vi "Dashboard custom_bartender.vi"() -> ()   [LabVIEW 2017]
uses:
  C:/Users/IMR Lab/Documents/LabVIEW Data/UniversalRobotsSDK_LABView/LabVIEW/Examples/LabVIEW10/UnderAutomation.UniversalRobots.dll
  UnderAutomation.UniversalRobots.dll
panel:
  out "\"3\"":bool
  out "\"2\"":bool
  out "\"1\"":bool
  out "UDP Loop Counter":i32
  out "UDP dataout":string
  in  "UDP":bool
  in  "stop":bool
  in  "TCP switch (server)":bool
  out "Rx":dbl
  out "Rz":dbl
  out "Ry":dbl
  out "Enabled":bool
  out "Port":i32
  in  "Move to particular posture":bool
  in  "Move to Zero position":bool
  out "Connected":bool
  in  "Robot IP(192.168.112.182)":string
  out "Connect error":errorcluster
  in  "Power on\nRelease brake":bool
  in  "Power off":bool
  in  "Connect":bool
  in  "Send script":bool
  in  "Script to execute":string
  out "Powered on":bool
  out "X":dbl
  out "Y":dbl
  out "Z":dbl
  out "License state":string
  # "movel(p[-0.0753945, -0.304532, 0.314608, -0.194623, 2.71667, -1.00228], a= 0.5, v=0.25)"
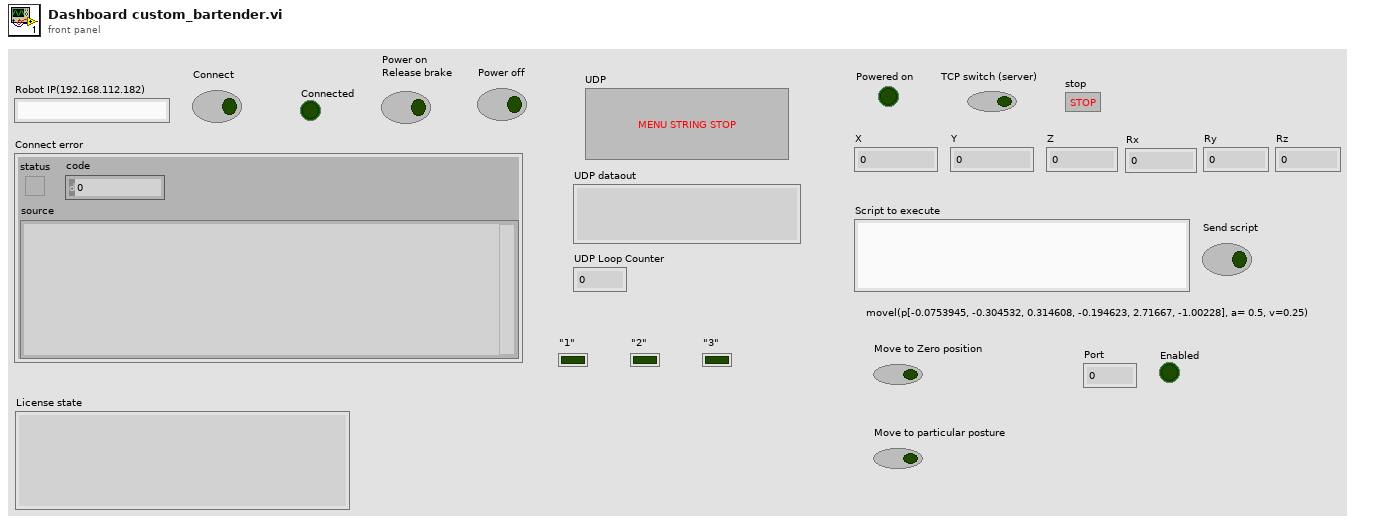
[diagram p1: front panel]
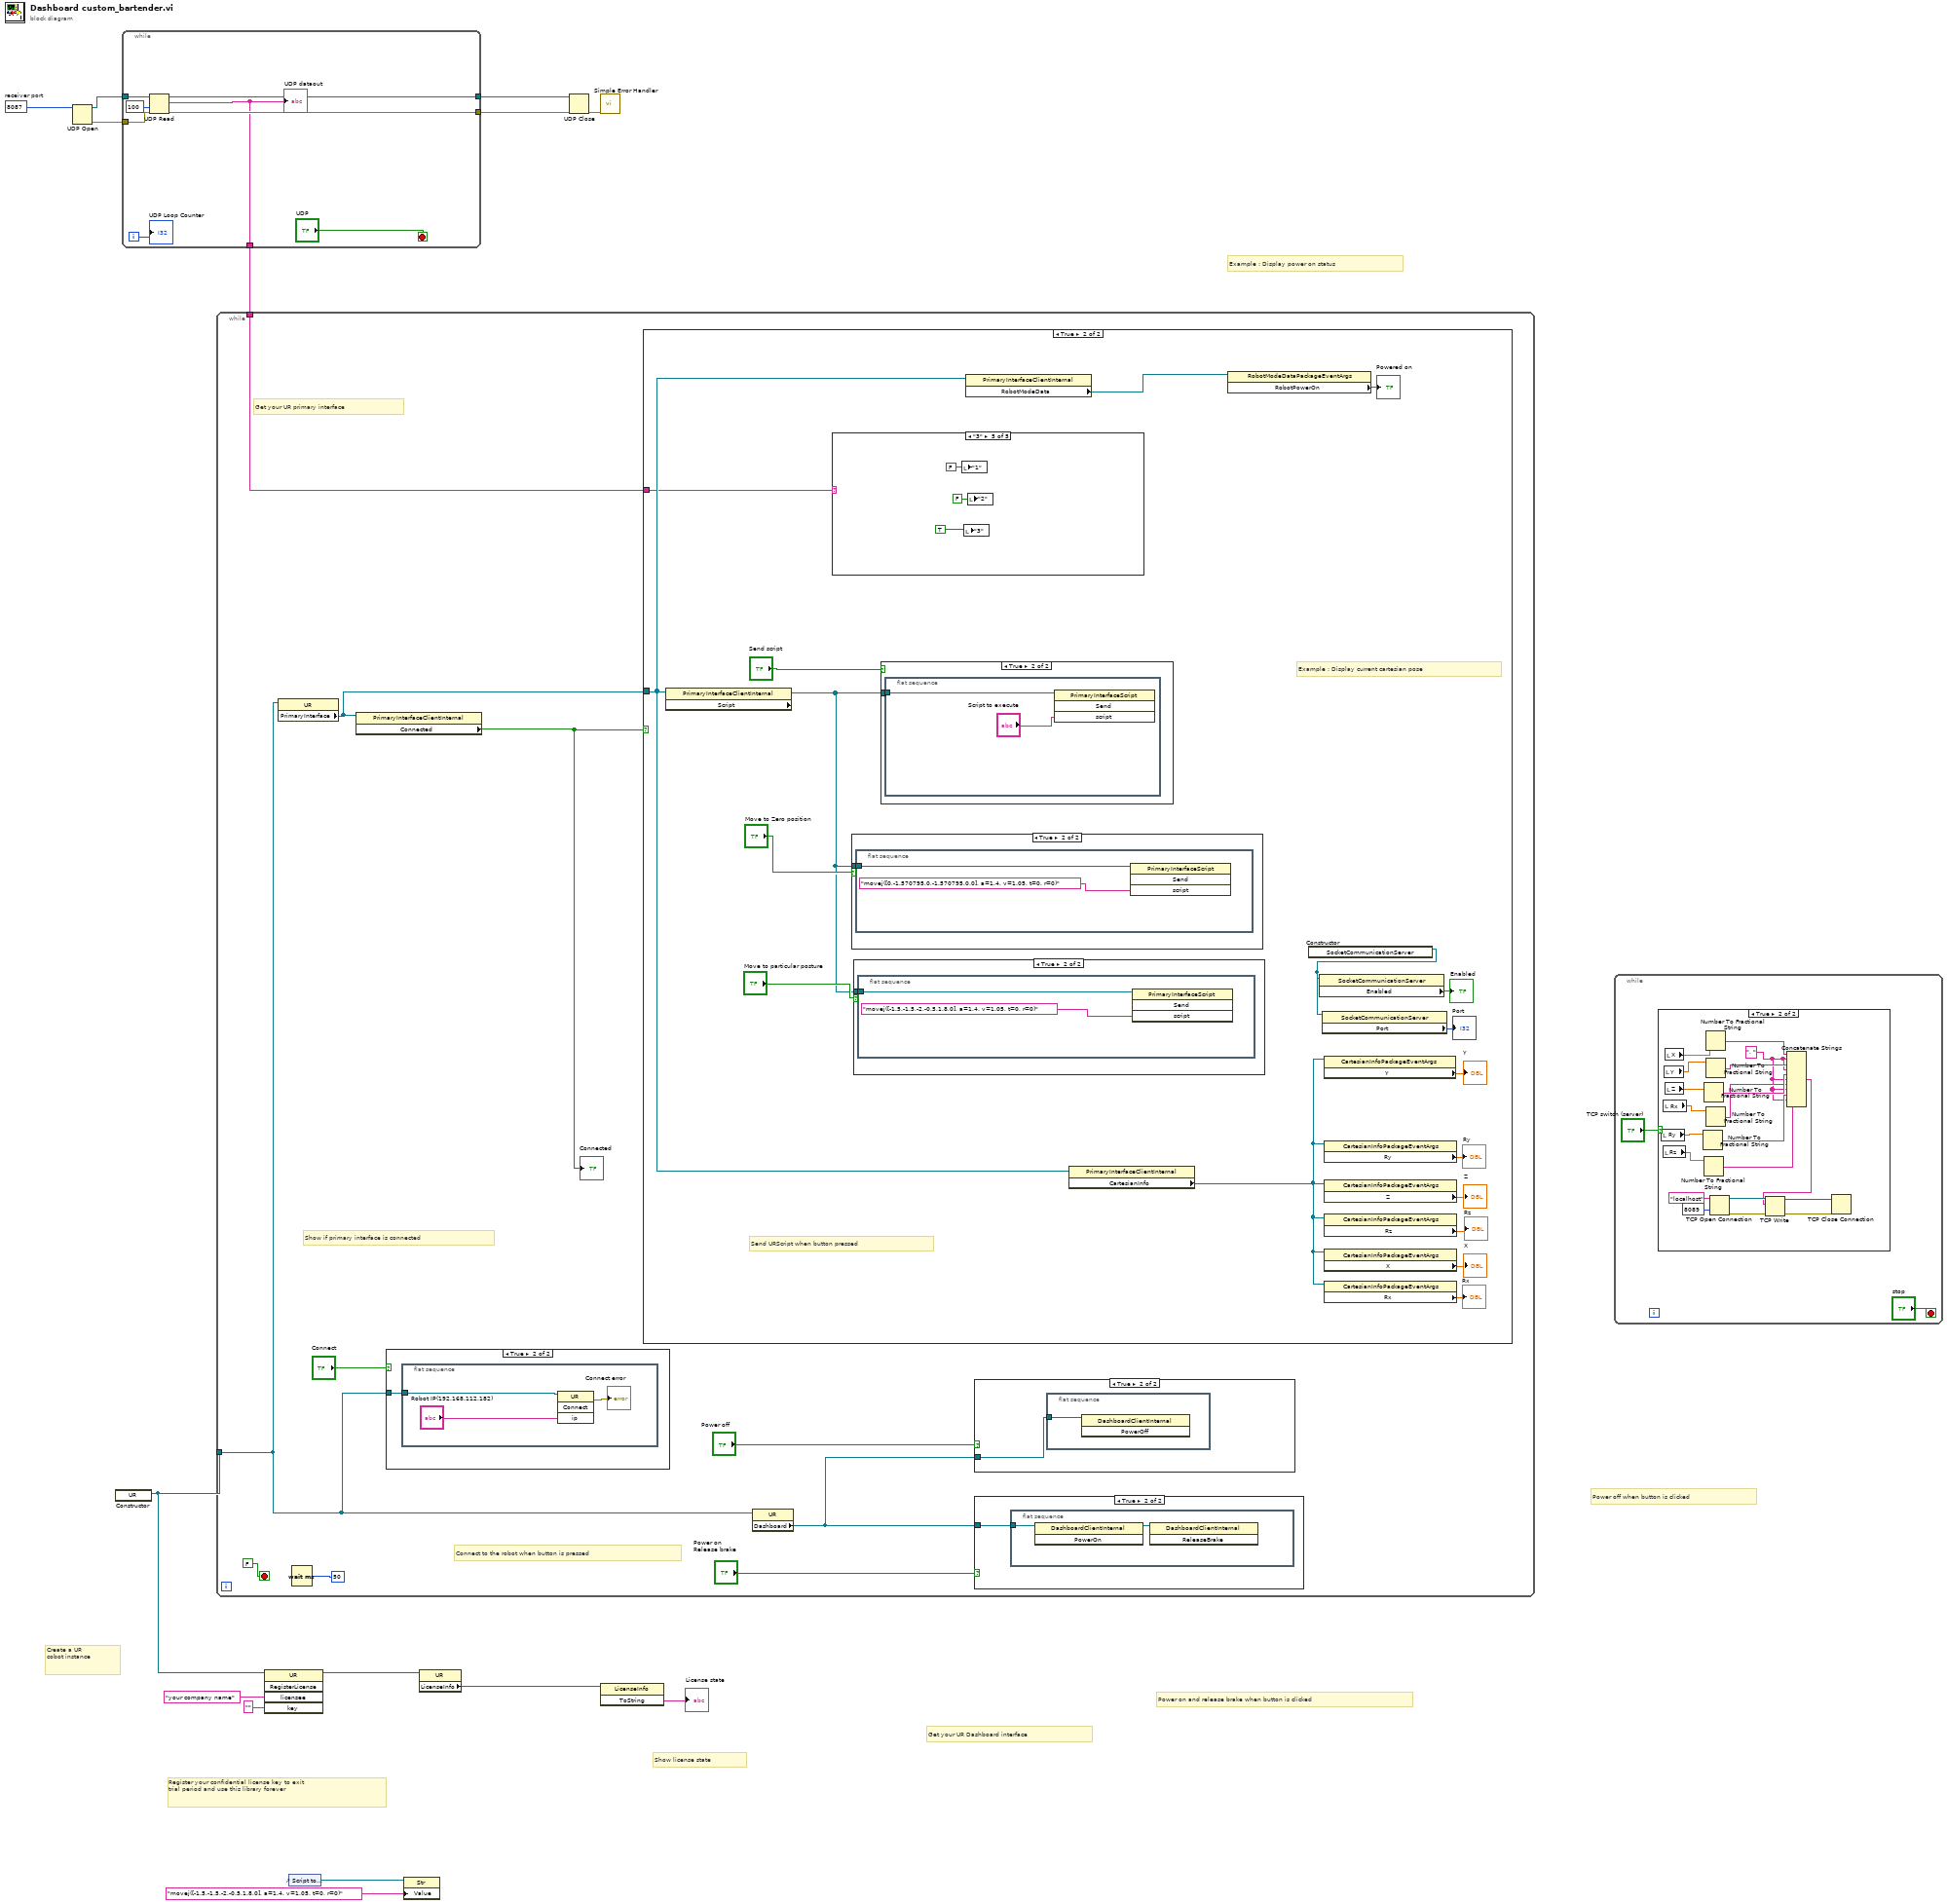
[diagram p0: block diagram]
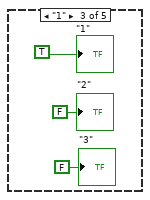
[diagram p6: hidden frame]
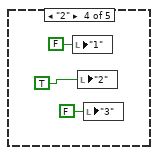
[diagram p7: hidden frame]
diagram:
  w7 = u16 8087  # receiver port
  # "Example : Display power on status"
  # "Create a UR\ncobot instance"
  # "Show license state"
  # "Register your confidential license key to exit\ntrial period and use this library forever"
  # "Power off when button is clicked"
  # "Power on and release brake when button is clicked"
  # "Get your UR Dashboard interface"
  n1 = UDP Open(11:w7) -> (port=w3:refnum<k16>, 0:w2:errorcluster)  [unwired: 4 in, 1 out]
  n2 = constructor class="UR"() -> (reference out=w10:refnum<k24>)  [unwired: 3 in, 2 out]
  n3 = while {
    tunnel: [w22] -> w5
    tunnel: [w21] -> w4
    tunnel: w3 -> [w20]
    tunnel: w2 -> [w19]
    tunnel: [w16] -> w1
    i -> [w18]
    stop <- "UDP" stop-if-true
    n4 = UDP Read(connection ID=w20, timeout ms (25000)=100, 8:w19) -> (data out=w16:string, error out=w21:errorcluster, 3:w22:refnum<k16>)  [unwired: 3 out]
    "UDP dataout" <- w16
    "UDP Loop Counter" <- w18
  }
  n5 = while {
    tunnel: w10 -> [w25]
    tunnel: w1 -> [w24]
    stop <- FALSE stop-if-true
    # "Connect to the robot when button is pressed"
    # "Show if primary interface is connected"
    # "Get your UR primary interface"
    n6 = property class="UR"(reference=w25) -> ("PrimaryInterface"=w28:refnum<k24>)  [unwired: 1 in, 2 out]
    n7 = Wait (ms)(milliseconds to wait=u32 50) -> ()  [unwired: 1 out]
    n8 = property class="PrimaryInterfaceClientInternal"(reference=w28) -> ("Connected"=w27:bool)  [unwired: 1 in, 2 out]
    "Connected" <- w27
    n9 = case shown="True" "Connect" {
      tunnel: w25 -> [_ w75]
      frame False {
      }
      frame True {
        n10 = flat-sequence {
          tunnel: w75 -> [w77]
          frame #0 {
            n11 = invoke class="UR" method="Connect"(reference=w77, "ip"="Robot IP(192.168.112.182)") -> (error out=→"Connect error":errorcluster)  [unwired: 2 in, 3 out]
          }
        }
      }
    }
    n12 = case shown="True" w27 {
      tunnel: w28 -> [_ w45]
      tunnel: w24 -> [_ w34]
      frame False {
      }
      frame True {
        # "Send URScript when button pressed"
        # "Example : Display current cartesian pose"
        n13 = property class="PrimaryInterfaceClientInternal"(reference=w45) -> ("Script"=w42:refnum<k24>)  [unwired: 1 in, 2 out]
        n14 = case shown="\"3\"" w34 {
          frame "False", Default {
          }
          frame "True" {
          }
          frame "1" {
            "\"1\"" <- TRUE
            "\"2\"" <- FALSE ("\"2\"")
            "\"3\"" <- FALSE ("\"3\"")
          }
          frame "2" {
            n15 = local write "\"1\""(FALSE ("\"1\"")) -> ()
            n16 = local write "\"2\""(TRUE) -> ()
            n17 = local write "\"3\""(FALSE ("\"3\"")) -> ()
          }
          frame "3" {
            n18 = local write "\"1\""(FALSE ("\"1\"")) -> ()
            n19 = local write "\"3\""(TRUE) -> ()
            n20 = local write "\"2\""(FALSE ("\"2\"")) -> ()
          }
        }
        n21 = case shown="True" "Move to Zero position" {
          tunnel: w42 -> [_ w64]
          frame False {
          }
          frame True {
            n22 = flat-sequence {
              tunnel: w64 -> [w66]
              frame #0 {
                n23 = invoke class="PrimaryInterfaceScript" method="Send"(reference=w66, "script"="movej([0,-1.570795,0,-1.570795,0,0], a=1.4, v=1.05, t=0, r=0)") -> ()  [unwired: 2 in, 4 out]
              }
            }
          }
        }
        n24 = case shown="True" "Move to particular posture" {
          tunnel: w42 -> [_ w61]
          frame False {
          }
          frame True {
            n25 = flat-sequence {
              tunnel: w61 -> [w63]
              frame #0 {
                n26 = invoke class="PrimaryInterfaceScript" method="Send"(reference=w63, "script"="movej([-1.5,-1.5,-2,-0.5,1.8,0], a=1.4, v=1.05, t=0, r=0)") -> ()  [unwired: 2 in, 4 out]
              }
            }
          }
        }
        n27 = case shown="True" "Send script" {
          tunnel: w42 -> [_ w67]
          frame False {
          }
          frame True {
            n28 = flat-sequence {
              tunnel: w67 -> [w69]
              frame #0 {
                n29 = invoke class="PrimaryInterfaceScript" method="Send"(reference=w69, "script"="Script to execute") -> ()  [unwired: 2 in, 4 out]
              }
            }
          }
        }
        n30 = property class="PrimaryInterfaceClientInternal"(reference=w45) -> ("RobotModeData"=w50:refnum<k24>)  [unwired: 1 in, 2 out]
        n31 = property class="PrimaryInterfaceClientInternal"(reference=w45) -> ("CartesianInfo"=w36:refnum<k24>)  [unwired: 1 in, 2 out]
        n32 = property class="RobotModeDataPackageEventArgs"(reference=w50) -> ("RobotPowerOn"=→"Powered on":bool)  [unwired: 1 in, 2 out]
        n33 = constructor class="SocketCommunicationServer"() -> (reference out=w41:refnum<k24>)  [unwired: 3 in, 2 out]
        n34 = property class="SocketCommunicationServer"(reference=w41) -> ("Enabled"=→"Enabled":bool)  [unwired: 1 in, 2 out]
        n35 = property class="SocketCommunicationServer"(reference=w41) -> ("Port"=→"Port":i32)  [unwired: 1 in, 2 out]
        n36 = property class="CartesianInfoPackageEventArgs"(reference=w36) -> ("Y"=→"Y":dbl)  [unwired: 1 in, 2 out]
        n37 = property class="CartesianInfoPackageEventArgs"(reference=w36) -> ("Ry"=→"Ry":dbl)  [unwired: 1 in, 2 out]
        n38 = property class="CartesianInfoPackageEventArgs"(reference=w36) -> ("Z"=→"Z":dbl)  [unwired: 1 in, 2 out]
        n39 = property class="CartesianInfoPackageEventArgs"(reference=w36) -> ("Rz"=→"Rz":dbl)  [unwired: 1 in, 2 out]
        n40 = property class="CartesianInfoPackageEventArgs"(reference=w36) -> ("X"=→"X":dbl)  [unwired: 1 in, 2 out]
        n41 = property class="CartesianInfoPackageEventArgs"(reference=w36) -> ("Rx"=→"Rx":dbl)  [unwired: 1 in, 2 out]
      }
    }
    n42 = property class="UR"(reference=w25) -> ("Dashboard"=w29:refnum<k24>)  [unwired: 1 in, 2 out]
    n43 = case shown="True" "Power off" {
      tunnel: w29 -> [_ w70]
      frame False {
      }
      frame True {
        n44 = flat-sequence {
          tunnel: w70 -> [w71]
          frame #0 {
            n45 = invoke class="DashboardClientInternal" method="PowerOff"(reference=w71) -> ()  [unwired: 2 in, 3 out]
          }
        }
      }
    }
    n46 = case shown="True" "Power on\nRelease brake" {
      tunnel: w29 -> [_ w72]
      frame False {
      }
      frame True {
        n47 = flat-sequence {
          tunnel: w72 -> [w74]
          frame #0 {
            n48 = invoke class="DashboardClientInternal" method="PowerOn"(reference=w74) -> (reference out=w73:refnum<k24>)  [unwired: 2 in, 2 out]
            n49 = invoke class="DashboardClientInternal" method="ReleaseBrake"(reference=w73) -> ()  [unwired: 2 in, 3 out]
          }
        }
      }
    }
  }
  n50 = invoke class="UR" method="RegisterLicense"(reference=w10, "licensee"="your company name", "key"="") -> (reference out=w12:refnum<k24>)  [unwired: 2 in, 4 out]
  n51 = control-ref of="Script to execute"() -> (w9:refnum<vi>)
  n52 = property class="Str"(reference=w9, "Value"="movej([-1.5,-1.5,-2,-0.5,1.8,0], a=1.4, v=1.05, t=0, r=0)") -> ()  [unwired: 1 in, 2 out]
  n53 = property class="UR"(reference=w12) -> ("LicenseInfo"=w11:refnum<k24>)  [unwired: 1 in, 2 out]
  n54 = UDP Close(connection ID=w5, 8:w4) -> (error out=w6:errorcluster)  [unwired: 1 out]
  n55 = call <vilib>:"Simple Error Handler.vi"("error in (no error)"=w6) -> ()  [unwired: 1 in, 8 out]
  n56 = invoke class="LicenseInfo" method="ToString"(reference=w11) -> ("ToString"=→"License state":string)  [unwired: 2 in, 2 out]
  n57 = while {
    stop <- "stop" stop-if-true
    n58 = case shown="True" "TCP switch (server)" {
      frame False {
      }
      frame True {
        w83 = ", "
        n59 = local read "Ry"() -> (w90:dbl)
        n60 = local read "Rz"() -> (w89:dbl)
        n61 = local read "Rx"() -> (w91:dbl)
        n62 = local read "Y"() -> (w93:dbl)
        n63 = local read "X"() -> (w94:dbl)
        n64 = local read "Z"() -> (w92:dbl)
        n65 = Number To Fractional String(number=w90) -> (F-format string=w84:string)  [unwired: 3 in]
        n66 = Number To Fractional String(number=w92) -> (F-format string=w86:string)  [unwired: 3 in]
        n67 = Number To Fractional String(number=w89) -> (F-format string=w82:string)  [unwired: 3 in]
        n68 = Number To Fractional String(number=w94) -> (F-format string=w88:string)  [unwired: 3 in]
        n69 = Number To Fractional String(number=w93) -> (F-format string=w87:string)  [unwired: 3 in]
        n70 = Number To Fractional String(number=w91) -> (F-format string=w85:string)  [unwired: 3 in]
        n71 = TCP Open Connection(address="localhost", remote port or service name=u16 8089) -> (connection ID=w98:refnum<k5>, error out=w97:errorcluster)  [unwired: 3 in]
        n72 = Concatenate Strings(w88, w83, w87, w83, w86, w83, w85, w83, w84, w83, w82) -> (w81:string)
        n73 = TCP Write(connection ID=w98, data in=w81, error in (no error)=w97) -> (connection ID out=w96:refnum<k5>, error out=w95:errorcluster)  [unwired: 1 in, 1 out]
        n74 = TCP Close Connection(connection ID=w96, error in (no error)=w95) -> ()  [unwired: 1 in, 2 out]
      }
    }
  }
